vi "Closest Points Array.vi"(8 "index":i32, 9 "Y in":dbl=359.5 format="%#_13g", 10 "X in":dbl=18.050867335505 format="%#_13g", 11 "All Lines":T1) -> (0 "Index on Line":i32, 3 "Array size":i32, 4 "element":cluster{"X":dbl, "Y":dbl, "Z":dbl})   [LabVIEW 2014]
uses:
  Libraries/Map Data Folder/All-Lines.ctl
  Libraries/Map Data Folder/LineCluster.ctl
  Libraries/Map Data Folder/LineConnection.ctl
  Libraries/Map Data Folder/Map Data.lvlib
panel:
  out "Index found?":bool
  out "Distance to nearest":dbl
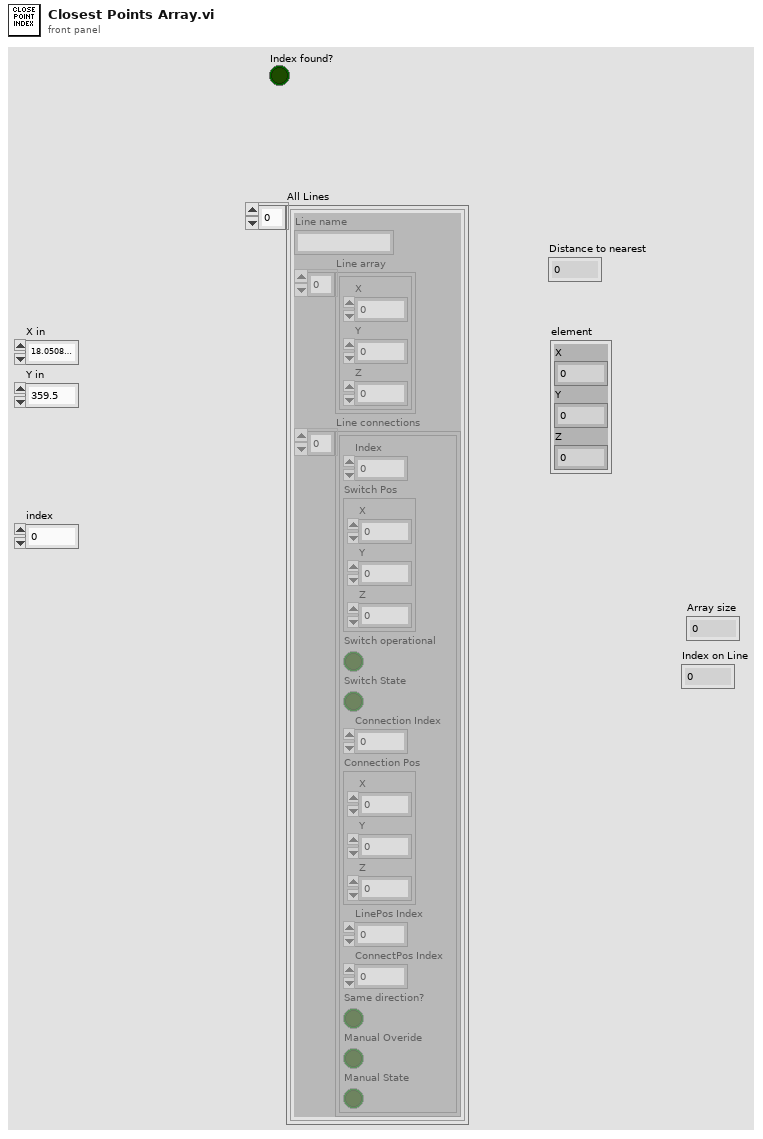
[diagram p1: front panel]
types:
  T1 = typedef "Map Data.lvlib/All-Lines.ctl" = T2[]
  T2 = typedef "Map Data.lvlib/LineCluster.ctl" = cluster{"Line name":string, "Line array":cluster{"X":dbl, "Y":dbl, "Z":dbl}[], "Line connections":T3[]}
  T3 = typedef "Map Data.lvlib/LineConnection.ctl" = cluster{"Index":i32, "Switch Pos":cluster{"X":dbl, "Y":dbl, "Z":dbl}, "Switch operational":bool, "Switch State":bool, "Connection Index":i32, "Connection Pos":cluster{"X":dbl, "Y":dbl, "Z":dbl}, "LinePos Index":i32, "ConnectPos Index":i32, "Same direction?":bool, "Manual Overide":bool, "Manual State":bool}
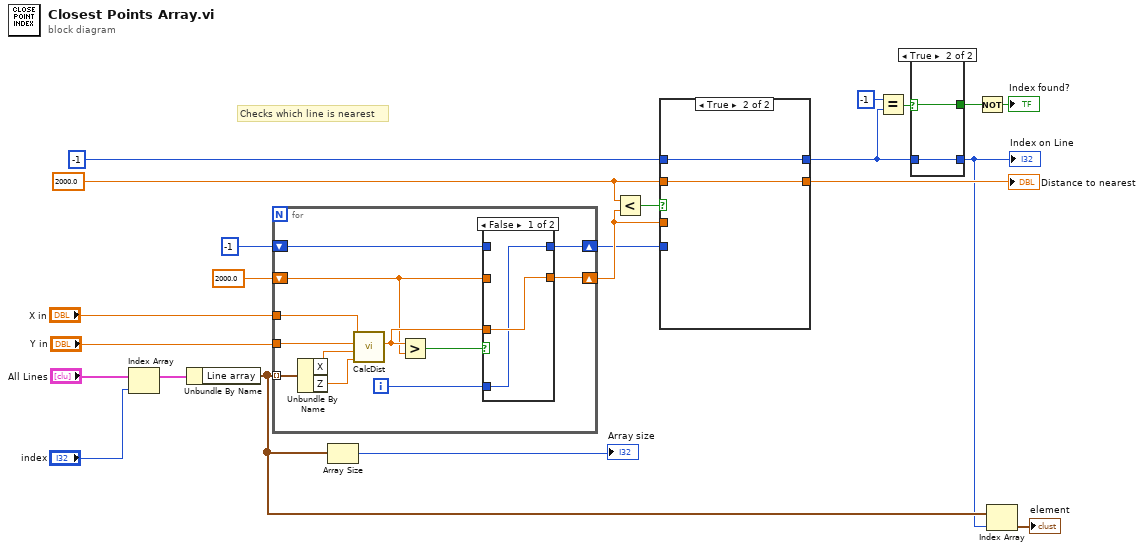
[diagram p0: block diagram]
diagram:
  w21 = 2000.0 ("Distance")
  # "Checks which line is nearest"
  n1 = Index Array(array="All Lines", index="index") -> (element=w9:T2)
  n2 = Unbundle By Name(w9) -> ("Line array"=w3:cluster{"X":dbl, "Y":dbl, "Z":dbl}[])
  n3 = for {
    tunnel: "X in" -> [w34]
    tunnel: w3 -> [w33] mode=indexing
    tunnel: "Y in" -> [w30]
    shift-right: [w27] -> w13
    shift-left: 2000.0 ("Distance") -> [w28]
    shift-right: [w25] -> w10
    shift-left: -1 -> [w26]
    i -> [w24]
    n4 = Unbundle By Name(w33) -> ("X"=w31:dbl, "Z"=w32:dbl)
    n5 = call "CalcDist.vi"("Y2"=w32, "X2"=w31, "Y1"=w30, "X1"=w34) -> ("Distance"=w29:dbl)  [unwired: 7 in]
    n6 = Greater?(x=w29, y=w28) -> (0:w23:bool)
    n7 = case shown="False" w23 {
      tunnel: w29 -> [w36 _]
      tunnel: [w36 w38] -> w27
      tunnel: w28 -> [_ w38]
      tunnel: w26 -> [_ w37]
      tunnel: w24 -> [w35 _]
      tunnel: [w35 w37] -> w25
      frame False {
      }
      frame True {
      }
    }
  }
  n8 = Array Size(array=w3) -> (size(s)=→"Array size":i32)
  n9 = Less?(x=w21, y=w13) -> (x < y?=w12:bool)
  n10 = case shown="True" w12 {
    tunnel: w13 -> [w40 _]
    tunnel: [w40 w42] -> w20
    tunnel: w21 -> [_ w42]
    tunnel: -1 -> [_ w41]
    tunnel: w10 -> [w39 _]
    tunnel: [w39 w41] -> w4
    frame False {
    }
    frame True {
    }
  }
  "Distance to nearest" <- w20
  n11 = Equal?(x=-1, y=w4) -> (x = y?=w15:bool)
  n12 = case shown="True" w15 {
    selector: w15 -> [w43 w46]
    tunnel: [w43 w46] -> w16
    tunnel: w4 -> [w44 w45]
    tunnel: [w44 w45] -> w2
    frame False {
    }
    frame True {
    }
  }
  "Index on Line" <- w2
  n13 = Not(x=w16) -> (.not. x?=→"Index found?":bool)
  n14 = Index Array(array=w3, index=w2) -> (element=→"element":cluster{"X":dbl, "Y":dbl, "Z":dbl})
